vi "AutoVisionDrive.vi"(6 "Distance (Inches)":dbl, 8 "error in":errorcluster, 9 "LeftDevRef":T1={"DeviceStatus"={"status"=FALSE, "code"=0, "source"=""}, "Type"=enum."PWM", "PWM"={"PWM Channel"=enum."PWM 1", "DeadBand"={"Name"="", "maxPositivePwm"=0, "minPositivePwm"=0, "centerPwm"=0, "maxNegativePwm"=0, "minNegativePwm"=0, "angularRange"=0}}, "CAN"={"Device Number"=0, "SetOutput VI Ref"=variant(enum8{"Percent VBus", "Current", "Speed", "Position", "Voltage"} enum."Percent VBus"), "GetOutput VI Ref"=variant(refnum<k1> refnum), "Enable VI Ref"=variant(dbl 12.0), "Disable VI Ref"=variant(enum8{"Percent VBus", "Speed", "Position", "Slave", "Unchanged / Invalid", "Voltage Compensation", "Current", "Motion Profile"} enum."Percent VBus"), "Data"=variant}, "Invert"=FALSE, "DIO PWM"={"PWM \"Enable\" Channel"=enum."Invalid", "DIOChannel"=enum."Invalid", "PWM Rate"=0.0}}, 10 "RightDevRef":T1={"DeviceStatus"={"status"=FALSE, "code"=0, "source"=""}, "Type"=enum."PWM", "PWM"={"PWM Channel"=enum."PWM 1", "DeadBand"={"Name"="", "maxPositivePwm"=0, "minPositivePwm"=0, "centerPwm"=0, "maxNegativePwm"=0, "minNegativePwm"=0, "angularRange"=0}}, "CAN"={"Device Number"=0, "SetOutput VI Ref"=variant(enum8{"Percent VBus", "Current", "Speed", "Position", "Voltage"} enum."Percent VBus"), "GetOutput VI Ref"=variant(refnum<k1> refnum), "Enable VI Ref"=variant(dbl 12.0), "Disable VI Ref"=variant(enum8{"Percent VBus", "Speed", "Position", "Slave", "Unchanged / Invalid", "Voltage Compensation", "Current", "Motion Profile"} enum."Percent VBus"), "Data"=variant}, "Invert"=FALSE, "DIO PWM"={"PWM \"Enable\" Channel"=enum."Invalid", "DIOChannel"=enum."Invalid", "PWM Rate"=0.0}}, 11 "DriveDevRef":T6={"DevStatus"={"status"=FALSE, "code"=0, "source"=""}, "Motors[]"=[], "Square Inputs"=FALSE, "Max Output"=1.0}) -> (0 "error out":errorcluster)   [LabVIEW 2017]
uses:
  <vilib>/Rock Robotics/WPI/RobotDrive/WPI_RobotDriveDevRef.ctl
  <vilib>/Rock Robotics/WPI/MotorControl/WPI_MotorControlDeviceRef.ctl
  <vilib>/Rock Robotics/WPI/MotorControl/WPI_MotorControlType.ctl
  <vilib>/Rock Robotics/SystemInterfaces/DIO/FPGA_DIOPWMChannel.ctl
  <vilib>/Rock Robotics/WPI/PWM/WPI_PWMDeadband.ctl
  <vilib>/Rock Robotics/SystemInterfaces/DIO/FPGA_DIOChannel.ctl
  <vilib>/Rock Robotics/Network Tables/NT Write Number.vi
  <vilib>/Rock Robotics/WPI/ThirdParty/Phoenix-LabVIEW/Motor Controller/Get/CTRE_Phoenix_MotorController_GetQuadratureData.vi
  <vilib>/Rock Robotics/WPI/RobotDrive/WPI_RobotDriveArcadeDrive_Standard(NoSaturation).vi
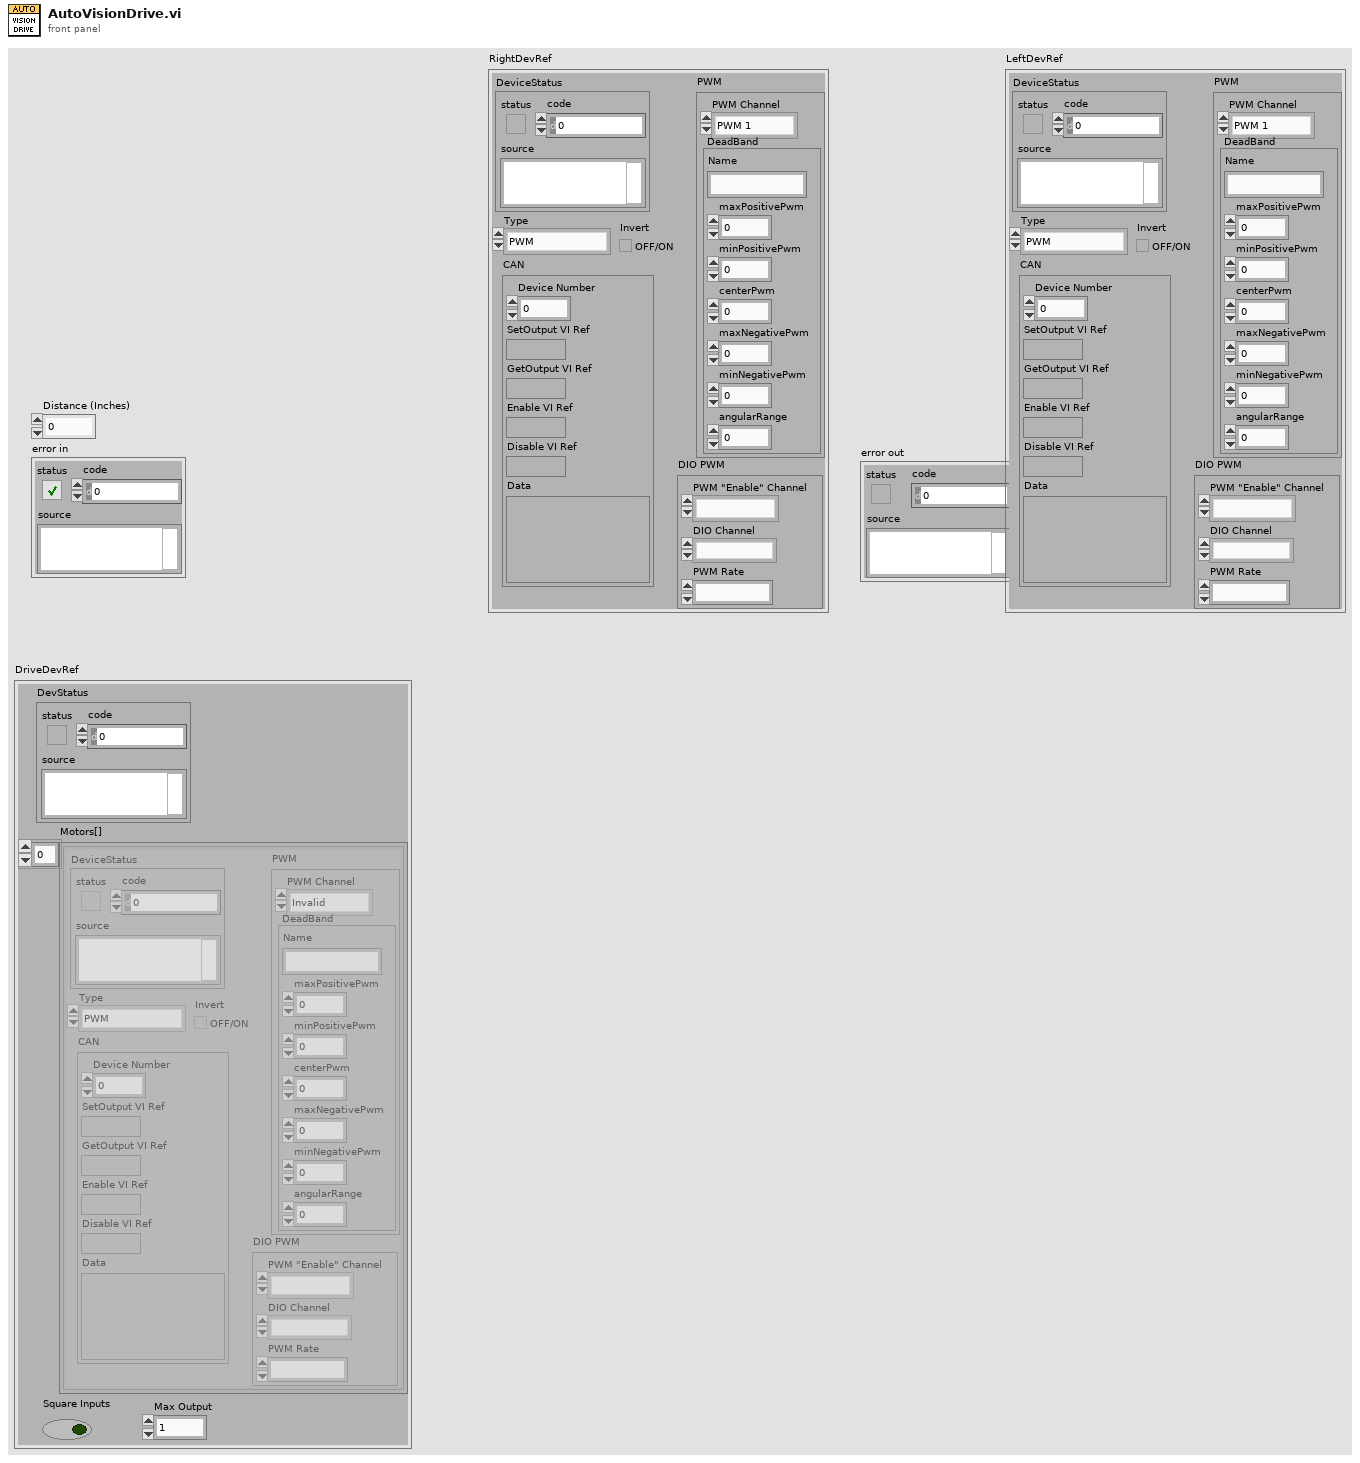
[diagram p1: front panel]
types:
  T1 = typedef "WPI_MotorControlDeviceRef.ctl" = cluster{"DeviceStatus":errorcluster, "Type":T2, "PWM":cluster{"PWM Channel":T3, "DeadBand":T4}, "CAN":cluster{"Device Number":u8, "SetOutput VI Ref":variant, "GetOutput VI Ref":variant, "Enable VI Ref":variant, "Disable VI Ref":variant, "Data":variant}, "Invert":bool, "DIO PWM":cluster{"PWM \"Enable\" Channel":T3, "DIOChannel":T5, "PWM Rate":dbl}}
  T2 = typedef "WPI_MotorControlType.ctl" = enum16{"PWM", "CAN", "DIO PWM"}
  T3 = typedef "FPGA_DIOPWMChannel.ctl" = enum8{"PWM 0", "PWM 1", "PWM 2", "PWM 3", "PWM 4", "PWM 5", "PWM 6", "PWM 7", "PWM 8", "PWM 9", "PWM MXP 0", "PWM MXP 1", "PWM MXP 2", "PWM MXP 3", "PWM MXP 4", "PWM MXP 5", "PWM MXP 6", "PWM MXP 7", "PWM MXP 8", "PWM MXP 9", "Invalid"}
  T4 = typedef "WPI_PWMDeadband.ctl" = cluster{"Name":string, "maxPositivePwm":i32, "minPositivePwm":i32, "centerPwm":i32, "maxNegativePwm":i32, "minNegativePwm":i32, "angularRange":u16}
  T5 = typedef "FPGA_DIOChannel.ctl" = enum8{"DIO 0", "DIO 1", "DIO 2", "DIO 3", "DIO 4", "DIO 5", "DIO 6", "DIO 7", "DIO 8", "DIO 9", "DIO MXP 0", "DIO MXP 1", "DIO MXP 2", "DIO MXP 3", "DIO MXP 4", "DIO MXP 5", "DIO MXP 6", "DIO MXP 7", "DIO MXP 8", "DIO MXP 9", "DIO MXP 10", "DIO MXP 11", "DIO MXP 12", "DIO MXP 13", "DIO MXP 14", "DIO MXP 15", "SPI Port CS1", "SPI Port CS2", "SPI Port CS3", "SPI Port MISO", "SPI Port MOSI", "Invalid"}
  T6 = typedef "WPI_RobotDriveDevRef.ctl" = cluster{"DevStatus":errorcluster, "Motors[]":T1[], "Square Inputs":bool, "Max Output":dbl}
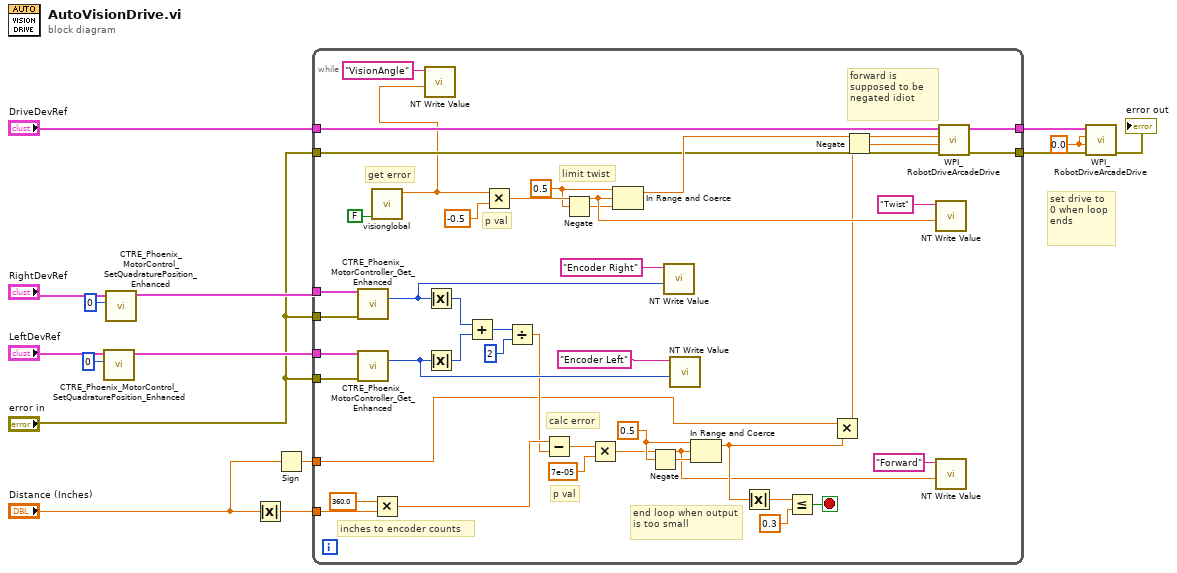
[diagram p0: block diagram]
diagram:
  w8 = 0.0 ("Y axis value")
  # "set drive to 0 when loop ends"
  n1 = call <vilib>:"CTRE_Phoenix_MotorControl_SetQuadraturePosition_Enhanced.vi"("New Position"=0, "PhoenixMotorControlDevRef"="LeftDevRef") -> ("PhoenixMotorControlDevRef"=w13:T1)  [unwired: 8 in, 1 out]
  n2 = call <vilib>:"CTRE_Phoenix_MotorControl_SetQuadraturePosition_Enhanced.vi"("New Position"=0, "PhoenixMotorControlDevRef"="RightDevRef") -> ("PhoenixMotorControlDevRef"=w14:T1)  [unwired: 8 in, 1 out]
  n3 = Absolute Value(x="Distance (Inches)") -> (abs(x)=w2:dbl)
  n4 = Sign(1:"Distance (Inches)") -> (0:w1:dbl)
  n5 = while {
    tunnel: w2 -> [w57]
    tunnel: w14 -> [w56]
    tunnel: w13 -> [w55]
    tunnel: "error in" -> [w47]
    tunnel: "error in" -> [w46]
    tunnel: "error in" -> [w45]
    tunnel: "DriveDevRef" -> [w44]
    tunnel: [w28] -> w10
    tunnel: [w27] -> w9
    tunnel: w1 -> [w19]
    stop <- w51 stop-if-true
    w22 = 0.5 ("upper limit")
    w24 = 0.5 ("upper limit")
    # "p val"
    # "calc error"
    # "end loop when output is too small"
    # "inches to encoder counts"
    # "limit twist"
    # "p val"
    # "get error"
    # "forward is supposed to be negated idiot"
    n6 = call-poly <vilib>:"CTRE_Phoenix_MotorController_Get_Enhanced.vi"("PhoenixMotorControlDevRef"=w56, "error in"=w47) -> ("Quadrature Position"=w43:i32)  [unwired: 10 in, 3 out]
    n7 = call-poly <vilib>:"CTRE_Phoenix_MotorController_Get_Enhanced.vi"("PhoenixMotorControlDevRef"=w55, "error in"=w45) -> ("Quadrature Position"=w40:i32)  [unwired: 10 in, 3 out]
    n8 = call "visionglobal.vi"("Set(T)/Get(F)"=FALSE) -> ("VisionAngle Out"=w16:dbl)  [unwired: 10 in]
    n9 = Multiply(x=360.0 ("convert"), y=w57) -> (x*y=w35:dbl)
    n10 = call-poly <vilib>:"NT Write Value.vi"("Numeric"=w16, "Name"="VisionAngle") -> ()  [unwired: 9 in, 1 out]
    n11 = Absolute Value(x=w43) -> (abs(x)=w54:i32)
    n12 = Absolute Value(x=w40) -> (abs(x)=w53:i32)
    n13 = Add(x=w54, y=w53) -> (x+y=w52:i32)
    n14 = Multiply(x=w16, y=-0.5 ("x")) -> (x*y=w39:dbl)
    n15 = Divide(x=w52, y=2) -> (x/y=w34:dbl)
    n16 = Subtract(x=w35, y=w34) -> (x-y=w31:dbl)
    n17 = Negate(x=w24) -> (-x=w25:dbl)
    n18 = Multiply(x=w31, y=7e-05) -> (x*y=w21:dbl)
    n19 = In Range and Coerce(upper limit=w24, x=w39, lower limit=w25) -> (coerced(x)=w48:dbl)  [unwired: 1 out]
    n20 = Negate(x=w22) -> (-x=w23:dbl)
    n21 = call-poly <vilib>:"NT Write Value.vi"("Numeric"=w43, "Name"="Encoder Right") -> ()  [unwired: 9 in, 1 out]
    n22 = call-poly <vilib>:"NT Write Value.vi"("Numeric"=w40, "Name"="Encoder Left") -> ()  [unwired: 9 in, 1 out]
    n23 = In Range and Coerce(upper limit=w22, x=w21, lower limit=w23) -> (coerced(x)=w26:dbl)  [unwired: 1 out]
    n24 = Absolute Value(x=w26) -> (abs(x)=w33:dbl)
    n25 = Less Or Equal?(x=w33, y=0.3) -> (x <= y?=w51:bool)
    n26 = Multiply(x=w19, y=w26) -> (x*y=w20:dbl)
    n27 = Negate(x=w20) -> (-x=w30:dbl)
    n28 = call-poly <vilib>:"NT Write Value.vi"("Numeric"=w39, "Name"="Twist") -> ()  [unwired: 9 in, 1 out]
    n29 = call-poly <vilib>:"NT Write Value.vi"("Numeric"=w21, "Name"="Forward") -> ()  [unwired: 9 in, 1 out]
    n30 = call-poly <vilib>:"WPI_RobotDriveArcadeDrive.vi"("error in (no error)"=w46, "Y axis value"=w30, "X axis value"=w48, "RobotDriveDevRef"=w44) -> ("error out"=w27:errorcluster, "RobotDriveDevRef"=w28:T6)  [unwired: 5 in, 1 out]
  }
  n31 = call-poly <vilib>:"WPI_RobotDriveArcadeDrive.vi"("error in (no error)"=w9, "Y axis value"=w8, "X axis value"=w8, "RobotDriveDevRef"=w10) -> ("error out"=→"error out":errorcluster)  [unwired: 5 in, 2 out]
